vi "Do.vi"(8 "error in (no error)":errorcluster, 10 "Actor in":refnum<class "Actor.lvclass">, 11 "Set Parameter Msg":refnum<class "Set Parameter Msg.lvclass">) -> (0 "error out":errorcluster, 2 "Actor out":refnum<class "Actor.lvclass">)   [LabVIEW 2014, in "Set Parameter Msg.lvclass"]
doc: "This VI delivers the message to the actor by calling the appropriate method(s) on the actor."
uses:
  Set Parameter Msg.lvclass
  <vilib>/ActorFramework/Actor/Actor.lvclass
  ParameterDevice.lvclass
  Set Parameter Msg.lvclass/Set Parameter Msg.ctl
  ExperimentService/Replay Msg.lvclass
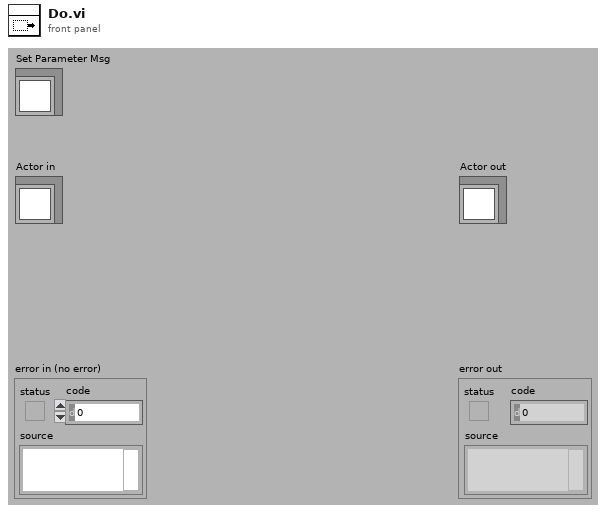
[diagram p1: front panel]
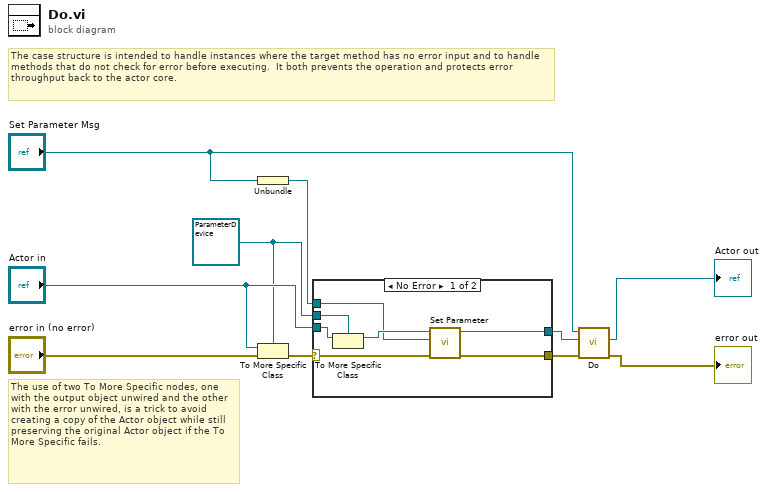
[diagram p0: block diagram]
diagram:
  w7 = refnum<class "ParameterDevice.lvclass"> refnum ("Actor in")
  # "The use of two To More Specific nodes, one with the output object unwired and the other with the error unwired, is a trick to avoid creating a copy of the Actor object while still preserving the original Actor object if the To More Specific fails."
  # "The case structure is intended to handle instances where the target method has no error input and to handle methods that do not check for error before executing.  It both prevents the operation and protects error throughput back to the actor core."
  n1 = Unbundle("Set Parameter Msg") -> (w6:refnum<class "AbstractData.lvclass">)
  n2 = To More Specific Class(target class=w7, reference="Actor in", error in="error in (no error)") -> (error out=w9:errorcluster)  [unwired: 1 out]
  n3 = case shown="No Error" w9 {
    selector: w9 -> [w15 w19]
    tunnel: [w17 w19] -> w3
    tunnel: [w16 w18] -> w4
    tunnel: "Actor in" -> [w14 w18]
    tunnel: w7 -> [w13 _]
    tunnel: w6 -> [w11 _]
    frame No Error {
      n4 = To More Specific Class(target class=w13, reference=w14) -> (specific class reference=w12:refnum<class "ParameterDevice.lvclass">)  [unwired: 1 in, 1 out]
      n5 = call-dynamic "Set Parameter.vi"("error in (no error)"=w15, "Parameter"=w11, "ParameterDevice in"=w12) -> ("error out"=w17:errorcluster, "ParameterDevice out"=w16:refnum<class "ParameterDevice.lvclass">)  [unwired: 7 in]
    }
    frame Error {
      # "If type check fails, pass the original object out again."
    }
  }
  n6 = call-parent "Do.vi"("error in (no error)"=w3, "Actor in"=w4, "Replay Message"="Set Parameter Msg") -> ("error out"=→"error out":errorcluster, "Actor out"=→"Actor out":refnum<class "Actor.lvclass">)  [unwired: 7 in]
